vi "Build File Path.vi"(8 "error in (no error)":errorcluster, 11 "Data Cluster in":T1) -> (0 "error out":errorcluster, 1 "appended path":path, 2 "Station ID":string, 3 "Data Cluster out":T1)   [LabVIEW 2018]
uses:
  Message Queue/Message Cluster.ctl
  Message Queue/GLDL Message Queue.lvlib
  Message Queue/All Message Queues.ctl
  controls/Connected Indicator.ctl
  controls/Output Indicator.ctl
  controls/Station ID Indicator.ctl
  controls/Disconnect Control.ctl
  controls/Download Control.ctl
  controls/Exit Control.ctl
  controls/Date Control.ctl
  controls/IP Phone Number Control.ctl
  controls/Reboot Control.ctl
  controls/Processing Loop State.ctl
  controls/GLDL UI Data.ctl
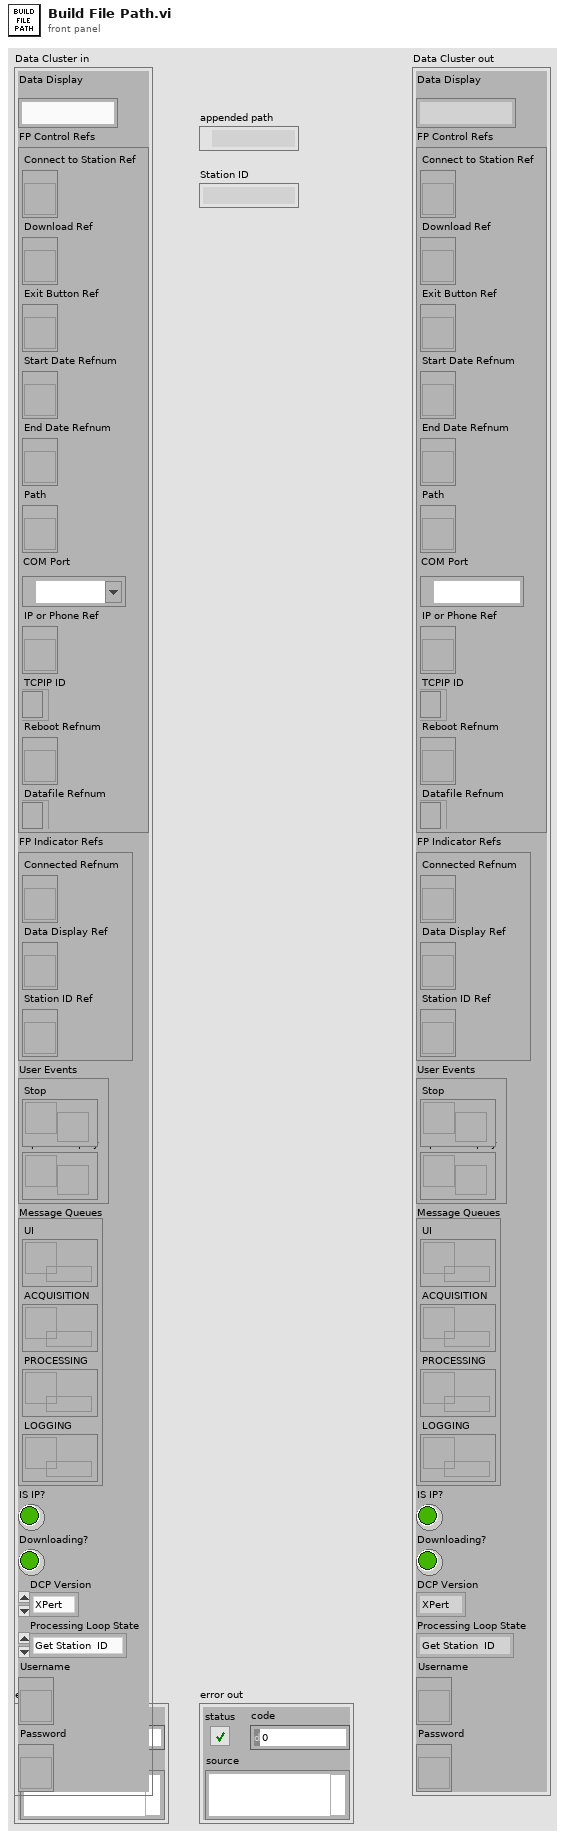
[diagram p1: front panel]
types:
  T1 = typedef "GLDL UI Data.ctl" = cluster{"Data Display":string, "FP Control Refs":cluster{"Connect to Station Ref":refnum<vi>, "Download Ref":refnum<vi>, "Exit Button Ref":refnum<vi>, "Start Date Refnum":refnum<vi>, "End Date Refnum":refnum<vi>, "Path":refnum<vi>, "COM Port":refnum<visa-resource-name>, "IP or Phone Ref":refnum<vi>, "TCPIP ID":refnum<k5>, "Reboot Refnum":refnum<vi>, "Datafile Refnum":refnum<file>}, "FP Indicator Refs":cluster{"Connected Refnum":refnum<vi>, "Data Display Ref":refnum<vi>, "Station ID Ref":refnum<vi>}, "User Events":cluster{"Stop":refnum<user-event>, "Update Display":refnum<user-event>}, "Message Queues":T2, "IS IP?":bool, "Downloading?":bool, "DCP Version":enum16{"XPert", "XPert2"}, "Processing Loop State":T3, "Username":refnum<vi>, "Password":refnum<vi>}
  T2 = typedef "GLDL Message Queue.lvlib/All Message Queues.ctl" = cluster{"UI":refnum<queue>, "ACQUISITION":refnum<queue>, "PROCESSING":refnum<queue>, "LOGGING":refnum<queue>}
  T3 = typedef "Processing Loop State.ctl" = enum16{"Get Station  ID", "Change Directory SD Card", "Change Directory Storage Card", "Downloading", "Idle in DL Directory"}
  T4 = typedef "Station ID Indicator.ctl" = string
  T5 = typedef "Date Control.ctl" = timestamp
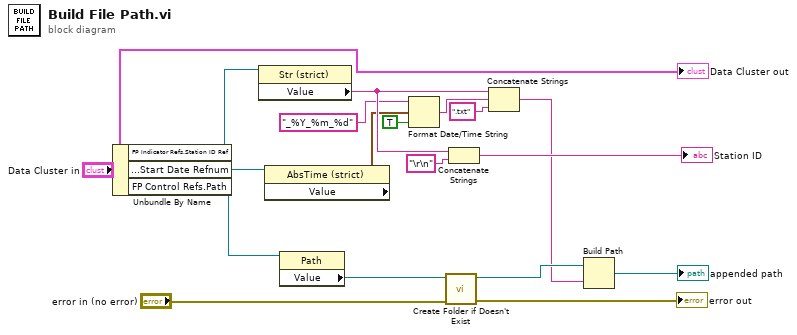
[diagram p0: block diagram]
diagram:
  n1 = Unbundle By Name("Data Cluster in") -> ("FP Indicator Refs.Station ID Ref"=w5:refnum<vi>, "FP Control Refs.Start Date Refnum"=w3:refnum<vi>, "FP Control Refs.Path"=w2:refnum<vi>)
  n2 = property class="Str (strict)"(reference=w5) -> ("Value"=w17:T4)  [unwired: 1 in, 2 out]
  n3 = property class="AbsTime (strict)"(reference=w3) -> ("Value"=w4:T5)  [unwired: 1 in, 2 out]
  n4 = property class="Path"(reference=w2) -> ("Value"=w13:path)  [unwired: 1 in, 2 out]
  n5 = Format Date/Time String(time format string (%c)="_%Y_%m_%d", seconds (now)=w4, UTC format=TRUE) -> (date/time string=w7:string)
  n6 = call "Create Folder if Doesn't Exist.vi"("error in (no error)"="error in (no error)", "Path In"=w13) -> ("error out"=→"error out":errorcluster, "Path Out"=w15:path)  [unwired: 8 in]
  n7 = Concatenate Strings(w17, "\r\n" ("time format string (%c)")) -> (→"Station ID":string)
  n8 = Concatenate Strings(w17, w7, ".txt" ("time format string (%c)")) -> (w9:string)
  n9 = Build Path(base path=w15, name or relative path=w9) -> (appended path=→"appended path":path)
  "Data Cluster out" <- "Data Cluster in"
